vi "Constants Map tester.vi"() -> ()   [LabVIEW 2013]
uses:
  Constants typedef V2.ctl
panel:
  in  "Read":string
  in  "Constants Array":T1[](array[typedef])
  out "Value 2":dbl
  in  "num buckets":i32=50
  out "Did it find it":bool
  in  "Value":dbl
  in  "Constant Name":string
  in  "error in (no error)":errorcluster
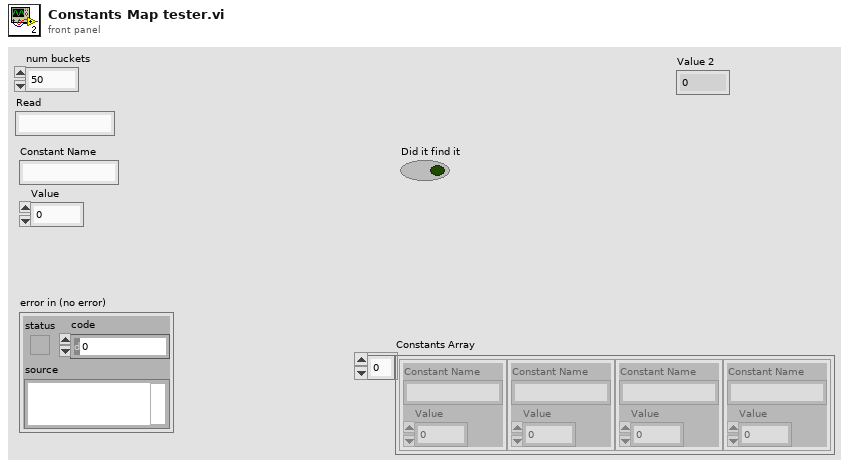
[diagram p1: front panel]
types:
  T1 = typedef "Constants typedef V2.ctl" = cluster{"Constant Name":string, "Value":dbl}
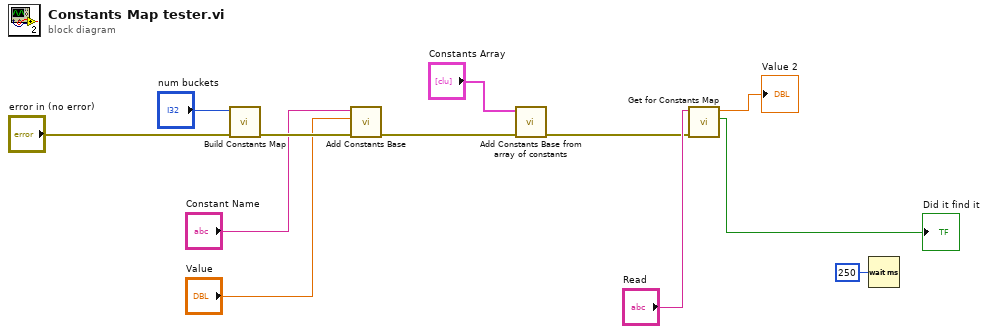
[diagram p0: block diagram]
diagram:
  n1 = call "Build Constants Map.vi"("error in (no error)"="error in (no error)", "num buckets"="num buckets") -> ("error out"=w9:errorcluster)  [unwired: 8 in, 1 out]
  n2 = call "Add Constants Base.vi"("error in (no error)"=w9, "Value"="Value", "Constant Name"="Constant Name") -> ("error out"=w2:errorcluster)  [unwired: 8 in]
  n3 = call "Add Constants Base from array of constants.vi"("error in (no error)"=w2, "Constants Array"="Constants Array") -> ("error out"=w1:errorcluster)  [unwired: 9 in]
  n4 = call "Get for Constants Map.vi"("error in (no error)"=w1, "Constant Name"="Read") -> ("Did it find it"=→"Did it find it":bool, "Value"=→"Value 2":dbl)  [unwired: 7 in, 1 out]
  n5 = Wait (ms)(milliseconds to wait=u32 250) -> ()  [unwired: 1 out]
